vi "Decompose LabVIEW Object - Child - Class Name Value.vi"() -> ()   [LabVIEW 2017, in "Composition.Tests.lvlib"]
uses:
  Composition.Tests.lvlib
  Classes/Child/Child.lvclass
  Composition/Composition.lvlib
  <vilib>/addons/_JKI Toolkits/Caraya/classes/Test/Test.lvclass
  <vilib>/addons/_JKI Toolkits/Caraya/classes/Assert/Assert.lvclass
panel:
  out "error out":errorcluster
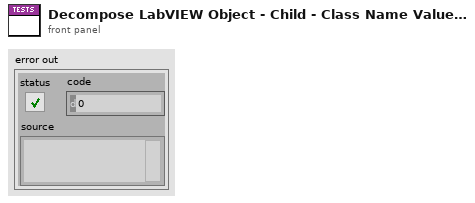
[diagram p1: front panel]
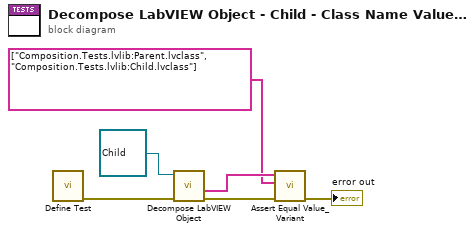
[diagram p0: block diagram]
diagram:
  n1 = call <vilib>:"Define Test.vi"() -> ("error out"=w3:errorcluster)  [unwired: 11 in]
  n2 = call "Decompose LabVIEW Object.vi"("error in (no error)"=w3, "LabVIEW Object"=refnum<class "Child.lvclass"> refnum ("Reflection.Tests.lvlib:Child.lvclass")) -> ("error out"=w5:errorcluster, "Class Names"=w2:string[])  [unwired: 6 in, 2 out]
  n3 = call <vilib>:"Assert Equal Value_Variant.vi"("error in (no error)"=w5, "Y"=string[] ["Composition.Tests.lvlib:Parent.lvclass", "Composition.Tests.lvlib:Child.lvclass"] ("Class Names"), "X"=w2) -> ("error out"=→"error out":errorcluster)  [unwired: 8 in]
